vi "PSTest.vi"   [LabVIEW 2018]
uses:
  ThirdParty/Keithley KE22xx Series/Keithley KE22xx Series.lvlib
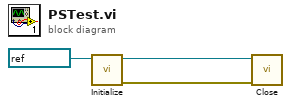
[diagram p0: block diagram]
diagram:
  n1 = call "Initialize.vi"("VISA resource name"=refnum<visa-resource-name> "COM1") -> ("error out"=w1:errorcluster, "VISA resource name out"=w2:refnum<visa-resource-name>)  [unwired: 9 in]
  n2 = call "Close.vi"("error in (no error)"=w1, "VISA resource name"=w2) -> ()  [unwired: 9 in, 1 out]
